vi "Color_Project.vi"() -> ()   [LabVIEW 2013]
uses:
  leitura de dados txt control.ctl
  <vilib>/Utility/file.llb/Write To Spreadsheet File (DBL).vi
panel:
  out "L*a*b* 3":dbl[](array[numeric])
  in  "C0":dbl min=0.0 max=1.0
  in  "RMix1":dbl[](array[numeric])
  in  "Selected RGB":string="0"
  in  "RMix2":dbl[](array[numeric])
  in  "Reflectance":dbl[](array[numeric])
  in  "Tab Control":T1(tab)
  in  "Create reflectance":bool
  in  "Nome da cor":string
  in  "SaveReflectance":bool
  out "Reflectance graph":cluster{"Value":dbl[], dbl[]}(graph) caption="Espectro de reflectância selecionado"
  in  "CalculateColor":bool
  in  "SelectReflectance":bool
  out "CMF graph":cluster{"X":dbl[], "Y":dbl[]}[](graph)
  in  "Select Illuminant":T2
  in  "Color Matching Function":string(combo)
  out "Iluminante Graph":cluster{"Value":dbl[], "Value":dbl[]}[](graph)
  in  "780nm":dbl(slide)=0.05 min=0.01 max=0.99 scale=0.0..1.0 scale format="%1.3f"
  in  "700nm":dbl(slide)=0.05 min=0.01 max=0.99 scale=0.0..1.0 scale format="%1.3f"
  in  "650nm":dbl(slide)=0.05 min=0.01 max=0.99 scale=0.0..1.0 scale format="%1.3f"
  in  "575nm":dbl(slide)=0.05 min=0.01 max=0.99 scale=0.0..1.0 scale format="%1.3f"
  in  "550nm":dbl(slide)=0.05 min=0.01 max=0.99 scale=0.0..1.0 scale format="%1.3f"
  in  "525nm":dbl(slide)=0.05 min=0.01 max=0.99 scale=0.0..1.0 scale format="%1.3f"
  in  "500nm":dbl(slide)=0.05 min=0.01 max=0.99 scale=0.0..1.0 scale format="%1.3f"
  in  "600nm":dbl(slide)=0.05 min=0.01 max=0.99 scale=0.0..1.0 scale format="%1.3f"
  in  "450nm":dbl(slide)=0.05 min=0.01 max=0.99 scale=0.0..1.0 scale format="%1.3f"
  in  "380nm":dbl(slide)=0.05 min=0.01 max=0.99 scale=0.0..1.0 scale format="%1.3f"
  out "Color":u32(colorbox)
  out "RGB":dbl[](array[numeric])
  out "XYZ":dbl[](array[numeric])
  out "RGB255":u32[](array[numeric]) caption="RGB"
  in  "Tab Control 3":enum32{"Misturar", "Estatísticas"}(tab)
  out "ColorRM":cluster{"Value":dbl[], "Mixtured colors":dbl[]}(graph) caption="Gráfico da reflectância das cores misturadas"
  in  "MixColors":bool
  in  "Selecione a concentração da cor 1":dbl(slide) scale=0.0..1.0 scale format="%#.4g"
  out "2000":dbl caption="Diferença: Cor 1 - Cor misturada"
  out "CD2-M":dbl caption="Diferença: Cor 2 - Cor misturada"
  out "L*a*b* MixedColor":dbl[](array[numeric]) caption="L*a*b* mixtura"
  out "L*a*b*":dbl[](array[numeric]) caption="L*a*b* cor 1"
  out "L*a*b* 2":dbl[](array[numeric]) caption="L*a*b* cor 2"
  out "Cor complementar":u32(colorbox)
  out "MixedColors":u32(colorbox) caption="Cor resultante"
  out "ColorR2":cluster{"Value":dbl[], "Mixtured colors":dbl[]}(graph) caption="Gráfico de reflectância da cor 2"
  out "ColorR1":cluster{"Value":dbl[], "Mixtured colors":dbl[]}(graph) caption="Gráfico de reflectância da cor 1"
  out "Color2":u32(colorbox) caption="Cor selecionada"
  out "Color1":u32(colorbox) caption="Cor selecionada"
  in  "SelectColor2":bool
  in  "SelectColor1":bool
  in  "Color Matching Function 2":string(combo) caption="Selecione o CMF"
  in  "SelectIlluminant2":T2 caption="Selecione o iluminante"
  out "Color1Complementar":u32(colorbox) caption="Cor complementar"
  out "Cor complementar  2":u32(colorbox) caption="Cor complementar"
  in  "SelectColor2":bool
  in  "SelectColor1":bool
  in  "Tab Control 2":enum32{"L*", "a*", "b*"}(tab)
  out "Componente L*":cluster{"X":dbl[], "L*a*b intermediary":dbl[]}(graph)
  out "Componente a*":cluster{"X":dbl[], "L*a*b intermediary":dbl[]}(graph)
  out "Componente b*":cluster{"X":dbl[], "L*a*b intermediary":dbl[]}(graph)
  in  "Color Matching Function 3":string(combo) caption="Selecione o CMF"
  in  "SelectIlluminant2 2":T2 caption="Selecione o iluminante"
  in  "Colors":u32[](array[colorbox])
  out "Espectros de reflectância referentes as cores intermediárias obtidas":cluster{"X":dbl[], "Y":dbl[]}[](graph)
  in  "MixByConcentration":bool
  in  "Mixed":dbl[](array[numeric])
  in  "MixByColorDifference":bool
  out "Color1 2":u32
  out "Color2 2":u32
  in  "C1":dbl=0.1 min=0.0 max=1.0
  in  "DeltaLabel":string[](array[string]) caption="Delta E"
  in  "ConcentrationLabel":string[](array[string]) caption="Concentração"
  out "teste":i32[](array[numeric])
  out "IL Table":string[][](array[string])
  out "ILCols":i32
  out "ILRows":i32
  out "Selected illuminant value":dbl[](array[numeric])
  out "Is CMF selected?":bool
  out "Is illuminant selected?":bool
  out "CMF Table":string[][](array[string])
  out "NeedInterpolation?":bool
  out "WhiteReference":i32[](array[numeric])
  out "Intepoled iluminants":dbl[][](array[numeric])
  out "Selected\nCMF":dbl[][](array[numeric])
  out "cmf Index":dbl
  out "CMFCols":i32
  out "CMFRows":i32
  out "LambdaInterval":dbl[](array[numeric])
  out "Selected illuminant index":dbl
  out "Selected illuminant NV":cluster{"Value":string, dbl[]}
  # "Primeira etapa - Seleção da iluminação desejada"
  # "Segunda etapa - Seleção do estímulo ocular do observador"
  # "Terceira etapa - Seleção ou criação de espectros de reflectância"
  # "Selecione o CMF"
  # "Selecione o iluminante"
  # "Etapa final - Calcular cor referente aos espectros"
  # "Sistema para criação de espectros de reflectância"
  # "Etapa básica - Seleção de iluminação e estímulos oculares"
  # "Etapa final - Calcular a mistura das cores e dosar a concentração da cor referência"
  # "Segunda etapa - Selecionar as cores desejadas para efetuar a mistura"
  # "Desvios de cor"
  # "Coordenadas de cor"
  # "Nesta seção serão avaliadas diferentes maneiras para misturas de cores:\n1 - Por variação de concentração\n2 - Por variação de desvio de cor"
  # "Análise de variação das componentes L*a*b* das cores geradas"
  # "Seleção de componentes"
  # "Seleção do tipo da mistura a ser efetuado"
  # "Representação das cores intermediárias gerada a partir\ndas misturas,e seus respectivos desvios e concentrações"
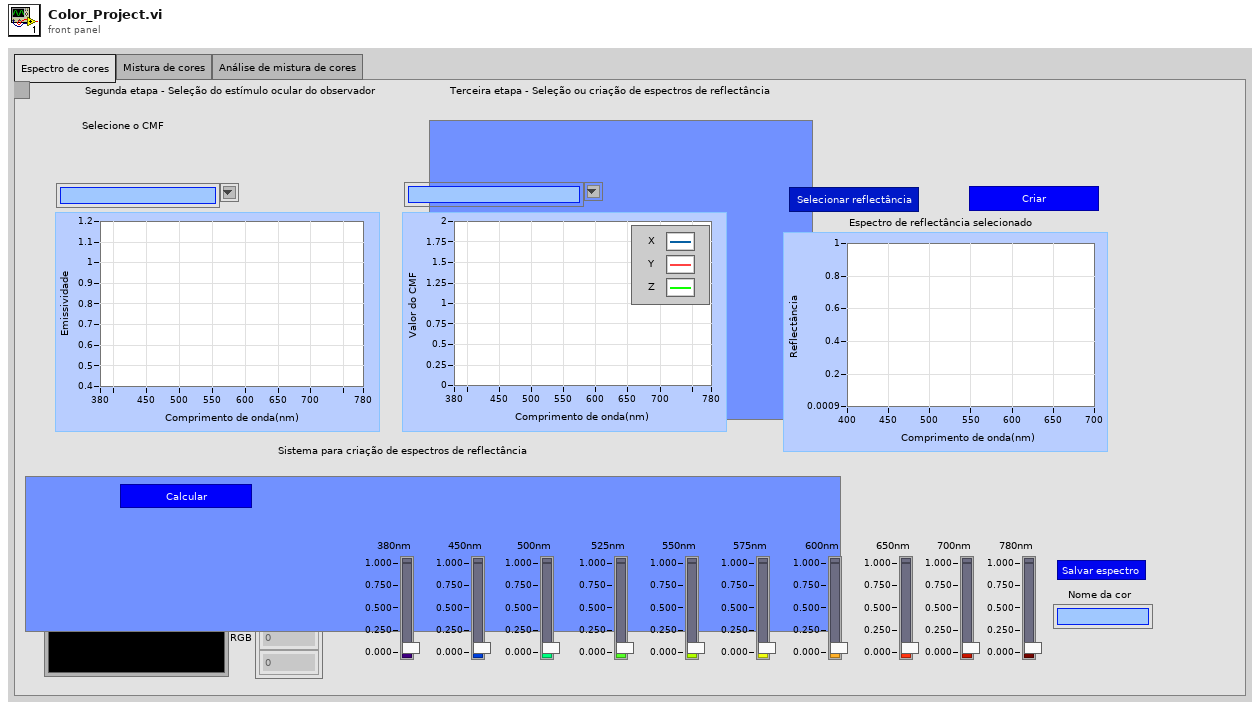
[diagram p1: front panel]
types:
  T1 = enum32{"Espectro de cores", "Mistura de cores", "Análise de mistura de cores"}
  T2 = typedef "leitura de dados txt control.ctl" = string
  T3 = cluster{"Value":cluster{"Value":string, dbl[]}, "Selected RGB":string, "Value":dbl[][]}
  T4 = cluster{"Color":u32, "RGB":dbl[], "L*a*b*":dbl[], "XYZ":dbl[]}
  T5 = cluster{cluster{i32[], dbl[]}, cluster{i32[], dbl[]}, cluster{i32[], dbl[]}}
  T6 = cluster{cluster{"X":dbl[], "L*a*b intermediary":dbl[]}, cluster{"X":dbl[], "L*a*b intermediary":dbl[]}, cluster{"X":dbl[], "L*a*b intermediary":dbl[]}}
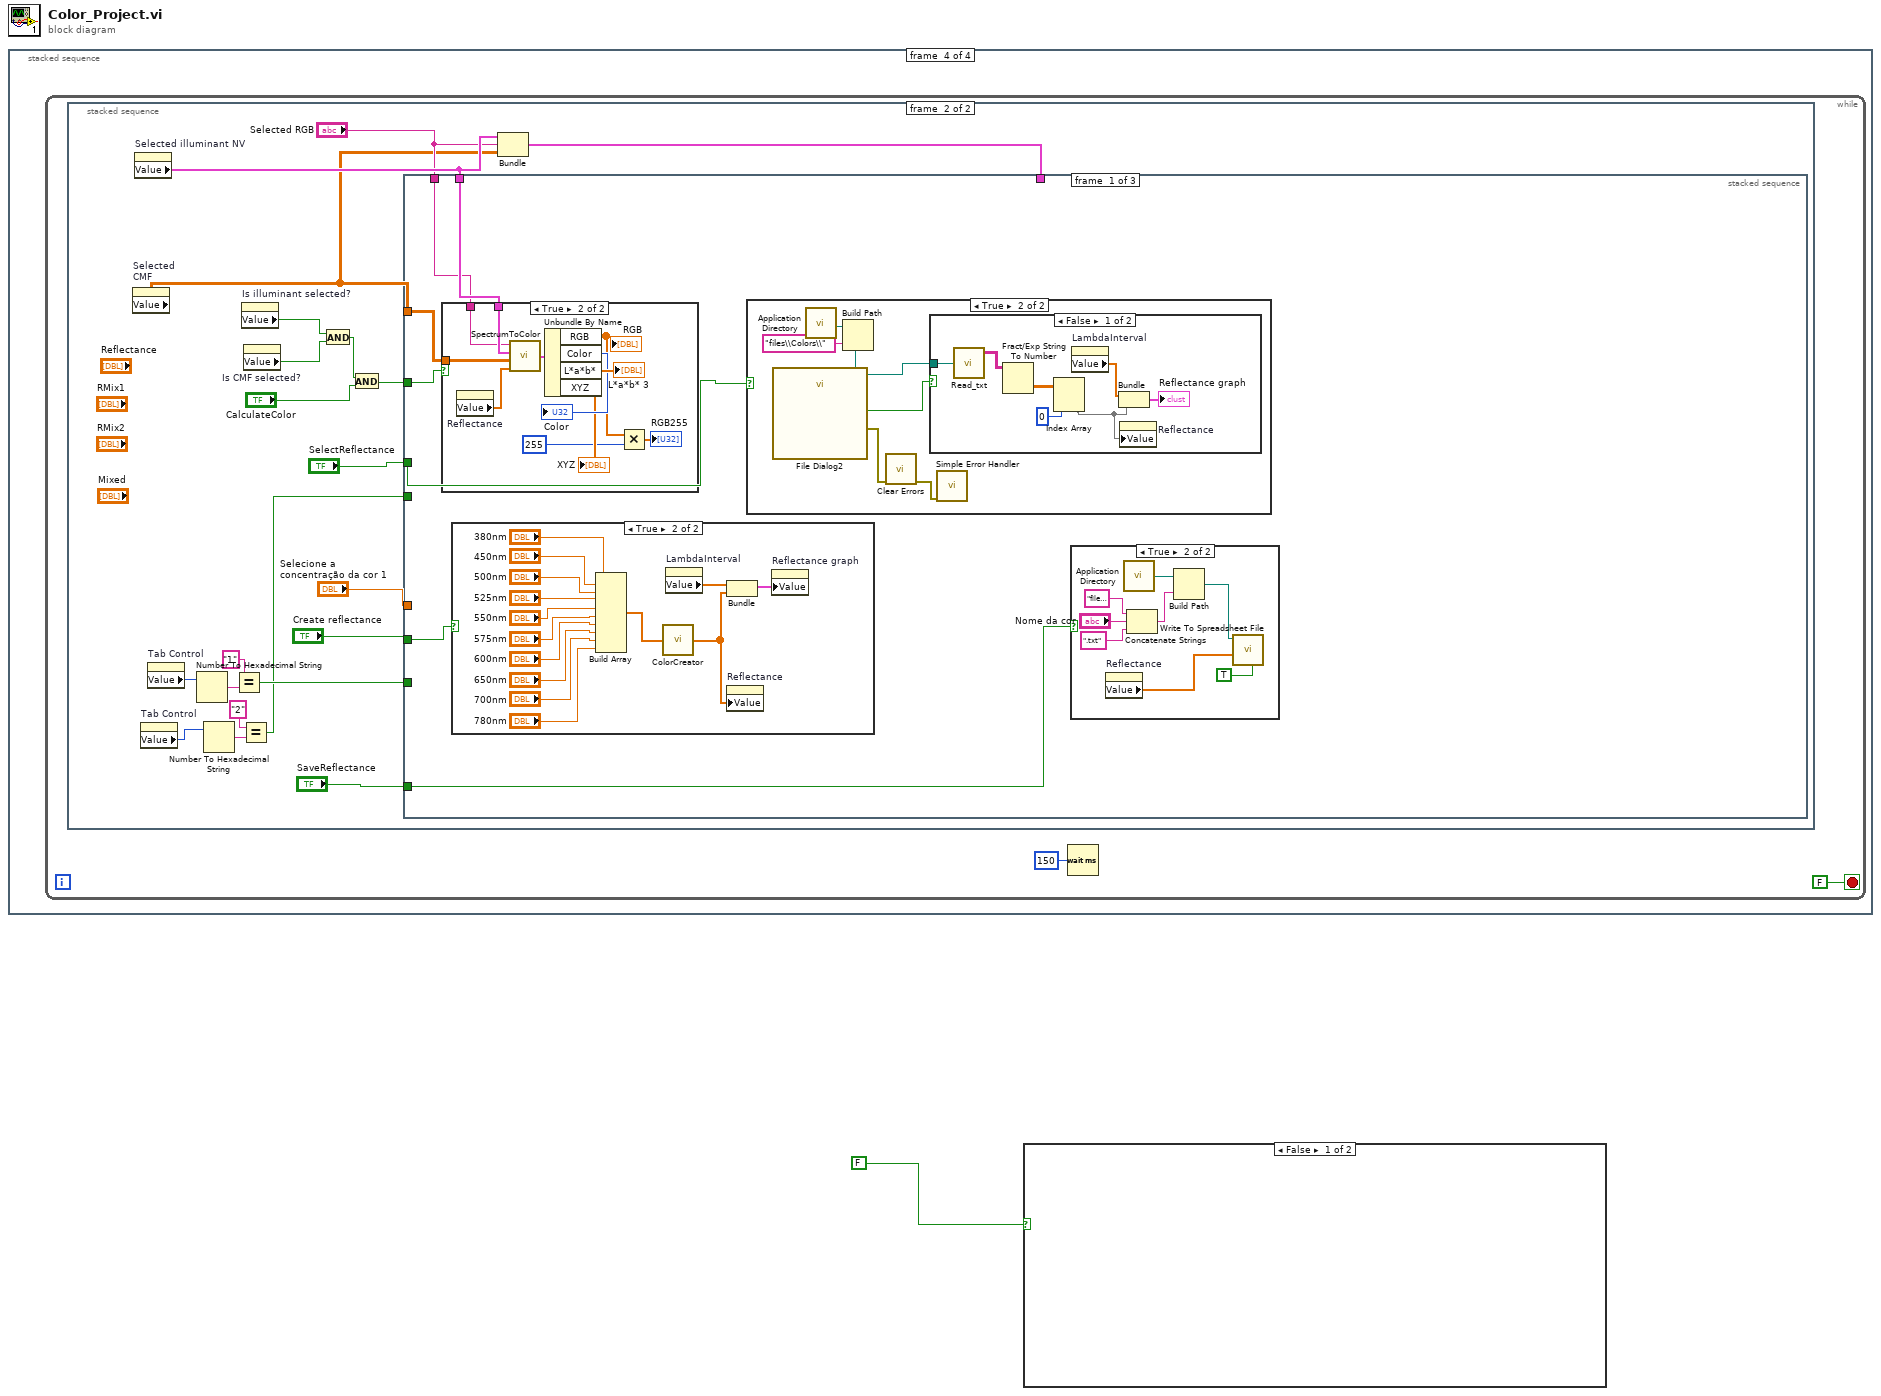
[diagram p0: block diagram]
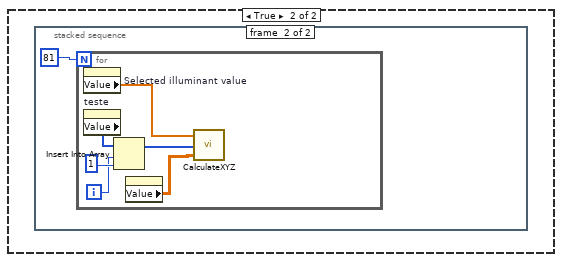
[diagram p2: hidden frame]
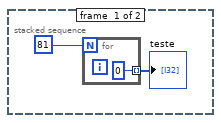
[diagram p3: hidden frame]
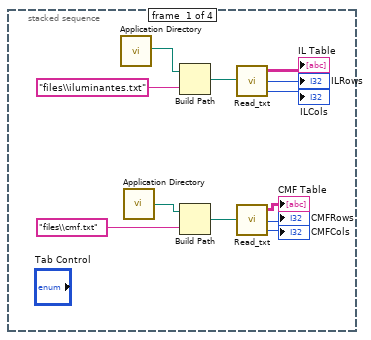
[diagram p4: hidden frame]
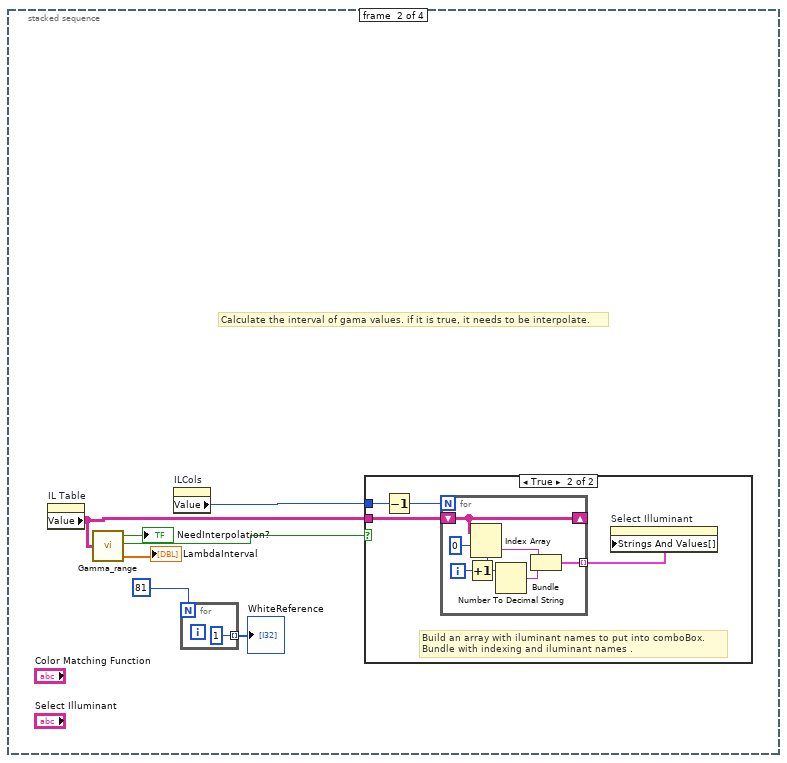
[diagram p5: hidden frame]
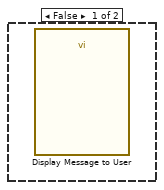
[diagram p6: hidden frame]
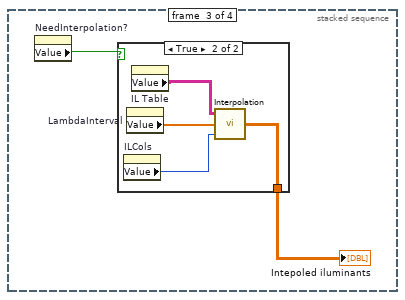
[diagram p7: hidden frame]
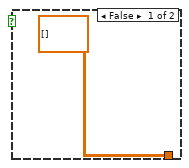
[diagram p8: hidden frame]
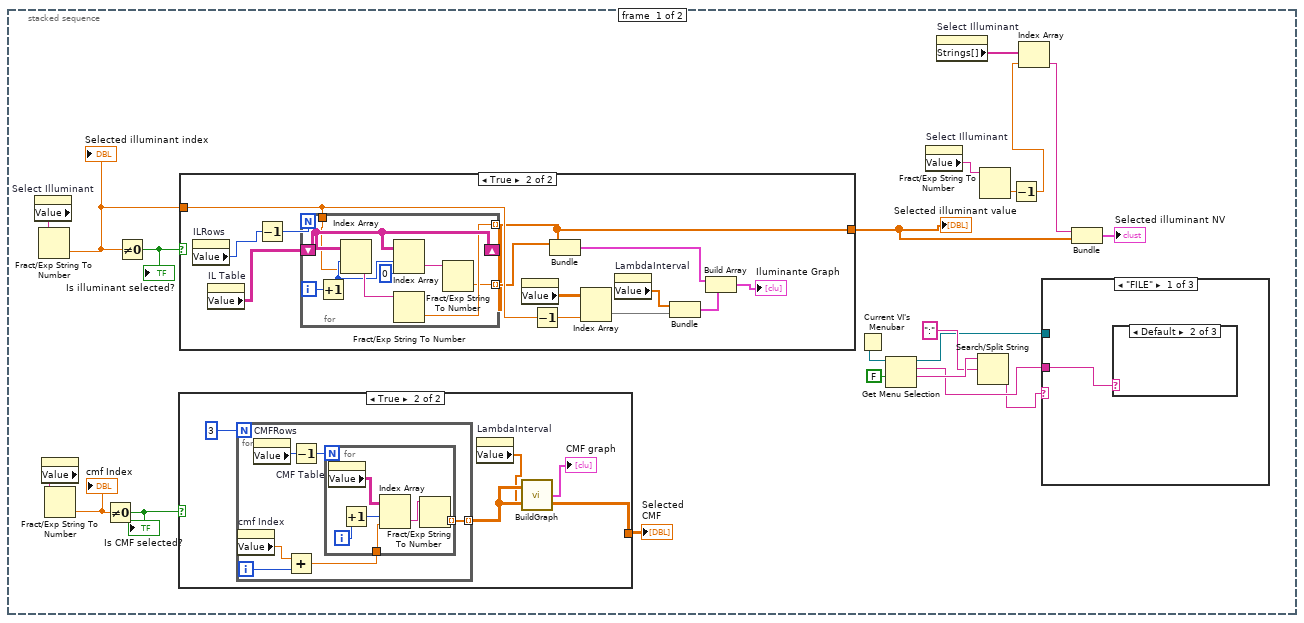
[diagram p9: hidden frame]
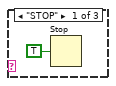
[diagram p10: hidden frame]
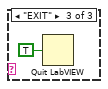
[diagram p11: hidden frame]
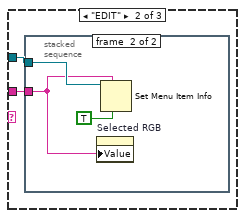
[diagram p12: hidden frame]
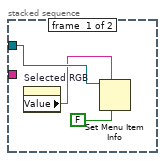
[diagram p13: hidden frame]
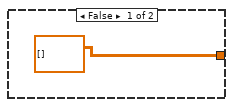
[diagram p15: hidden frame]
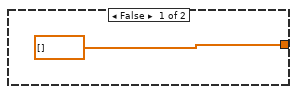
[diagram p16: hidden frame]
diagram:
  n1 = stacked-sequence {
    frame #0 {
      n2 = call <vilib>:"Application Directory.vi"() -> ("Application Directory"=w3:path)
      n3 = call <vilib>:"Application Directory.vi"() -> ("Application Directory"=w2:path)
      n4 = Build Path(base path=w3, name or relative path="files\\iluminantes.txt") -> (appended path=w5:path)
      n5 = Build Path(base path=w2, name or relative path="files\\cmf.txt") -> (appended path=w4:path)
      n6 = call "Read_txt.vi"("file path (dialog if empty)"=w5) -> ("Elements"=→"IL Table":string[][], "Rows"=→"ILRows":i32, "Cols"=→"ILCols":i32)
      n7 = call "Read_txt.vi"("file path (dialog if empty)"=w4) -> ("Elements"=→"CMF Table":string[][], "Rows"=→"CMFRows":i32, "Cols"=→"CMFCols":i32)
    }
    frame #1 {
      # "Calculate the interval of gama values. if it is true, it needs to be interpolate."
      n8 = property on="IL Table" class="Arr (strict)"() -> ("Value"=w15:string[][])  [unwired: 2 in, 2 out]
      n9 = call "Gamma_range.vi"("Illuminant Table"=w15) -> ("Interpolate"=→"NeedInterpolation?":bool, "In range?"=w17:bool, "GammaInterval"=→"LambdaInterval":dbl[])
      n10 = property on="ILCols" class="DigNum (strict)"() -> ("Value"=w18:i32)  [unwired: 2 in, 2 out]
      n11 = for {
        N: 81 -> [_]
        tunnel: [1] -> w19 mode=indexing
      }
      "WhiteReference" <- w19
      n12 = case shown="True" w17 {
        tunnel: w15 -> [_ w21]
        tunnel: w18 -> [_ w22]
        frame False {
          n13 = call "Display Message to User"() -> ()  [unwired: 10 in, 2 out]
        }
        frame True {
          # "Build an array with iluminant names to put into comboBox.\nBundle with indexing and iluminant names ."
          n14 = Decrement(x=w22) -> (x-1=w24:i32)
          n15 = for {
            N: w24 -> [_]
            shift-right: [w29] -> _
            shift-left: w21 -> [w29]
            tunnel: [w25] -> w23 mode=indexing
            i -> [w31]
            n16 = Increment(x=w31) -> (x+1=w28:i32)
            n17 = Index Array(array=w29, index (row)=0, index (col)=w28) -> (element=w26:string)
            n18 = Number To Decimal String(number=w28) -> (decimal integer string=w27:string)  [unwired: 1 in]
            n19 = Bundle("String"=w26, w27) -> (w25:cluster{"String":string, string})  [unwired: 1 in]
          }
          n20 = property on="Select Illuminant" class="CmbBox (strict)"("Strings And Values[]"=w23) -> ()  [unwired: 2 in, 2 out]
        }
      }
    }
    frame #2 {
      n21 = property on="NeedInterpolation?" class="Bool (strict)"() -> ("Value"=w34:bool)  [unwired: 2 in, 2 out]
      n22 = case shown="True" w34 {
        tunnel: [dbl[][] [] w38] -> w33
        frame False {
        }
        frame True {
          n23 = property on="ILCols" class="DigNum (strict)"() -> ("Value"=w36:i32)  [unwired: 2 in, 2 out]
          n24 = property on="LambdaInterval" class="Arr (strict)"() -> ("Value"=w39:dbl[])  [unwired: 2 in, 2 out]
          n25 = property on="IL Table" class="Arr (strict)"() -> ("Value"=w37:string[][])  [unwired: 2 in, 2 out]
          n26 = call "Interpolation.vi"("Number of Columns"=w36, "Lambda Interval"=w39, "Illuminants"=w37) -> ("Interpolated"=w38:dbl[][])
        }
      }
      "Intepoled iluminants" <- w33
    }
    frame #3 {
      n27 = while {
        stop <- FALSE stop-if-true
        n28 = stacked-sequence {
          frame #0 {
            n29 = property on="Select Illuminant" class="CmbBox (strict)"() -> ("Value"=w58:T2)  [unwired: 2 in, 2 out]
            n30 = Fract/Exp String To Number(string=w58) -> (number=w57:dbl)  [unwired: 3 in, 1 out]
            "Selected illuminant index" <- w57
            n31 = property on="Color Matching Function" class="CmbBox"() -> ("Value"=w60:string)  [unwired: 2 in, 2 out]
            n32 = Fract/Exp String To Number(string=w60) -> (number=w61:dbl)  [unwired: 3 in, 1 out]
            "cmf Index" <- w61
            n33 = Not Equal To 0?(x=w61) -> (x != 0?=w59:bool)
            "Is CMF selected?" <- w59
            n34 = Not Equal To 0?(x=w57) -> (x != 0?=w62:bool)
            "Is illuminant selected?" <- w62
            n35 = case shown="True" w59 {
              tunnel: [dbl[][] [] w77] -> w56
              frame False {
              }
              frame True {
                n36 = for {
                  N: 3 -> [_]
                  tunnel: [w81] -> w77 mode=indexing
                  i -> [w83]
                  n37 = property on="cmf Index" class="DigNum (strict)"() -> ("Value"=w84:dbl)  [unwired: 2 in, 2 out]
                  n38 = property on="CMFRows" class="DigNum (strict)"() -> ("Value"=w80:i32)  [unwired: 2 in, 2 out]
                  n39 = Add(x=w84, y=w83) -> (x+y=w82:dbl)
                  n40 = Decrement(x=w80) -> (x-1=w79:i32)
                  n41 = for {
                    N: w79 -> [_]
                    tunnel: w82 -> [w89]
                    tunnel: [w85] -> w81 mode=indexing
                    i -> [w88]
                    n42 = property on="CMF Table" class="Arr (strict)"() -> ("Value"=w90:string[][])  [unwired: 2 in, 2 out]
                    n43 = Increment(x=w88) -> (x+1=w87:i32)
                    n44 = Index Array(array=w90, index (row)=w87, index (col)=w89) -> (element=w86:string)
                    n45 = Fract/Exp String To Number(string=w86) -> (number=w85:dbl)  [unwired: 3 in, 1 out]
                  }
                }
                n46 = property on="LambdaInterval" class="Arr (strict)"() -> ("Value"=w76:dbl[])  [unwired: 2 in, 2 out]
                n47 = call "BuildGraph.vi"("X"=w76, "Y"=w77) -> ("Graph"=→"CMF graph":cluster{"X":dbl[], "Y":dbl[]}[])
              }
            }
            "Selected\nCMF" <- w56
            n48 = case shown="True" w62 {
              tunnel: w57 -> [_ w101]
              tunnel: [dbl[] [] w95] -> w55
              frame False {
              }
              frame True {
                n49 = property on="ILRows" class="DigNum (strict)"() -> ("Value"=w94:i32)  [unwired: 2 in, 2 out]
                n50 = property on="IL Table" class="Arr (strict)"() -> ("Value"=w93:string[][])  [unwired: 2 in, 2 out]
                n51 = Decrement(x=w94) -> (x-1=w104:i32)
                n52 = for {
                  N: w104 -> [_]
                  shift-right: [w112] -> _
                  shift-left: w93 -> [w112]
                  tunnel: w101 -> [w105]
                  tunnel: [w107] -> w95 mode=indexing
                  tunnel: [w106] -> w97 mode=indexing
                  i -> [w113]
                  n53 = Increment(x=w113) -> (x+1=w108:i32)
                  n54 = Index Array(array=w112, index (row)=w108, index (col)=w105) -> (element=w109:string)
                  n55 = Index Array(array=w112, index (row)=w108, index (col)=0 ("disabled index (col)")) -> (element=w110:string)
                  n56 = Fract/Exp String To Number(string=w109) -> (number=w107:dbl)  [unwired: 3 in, 1 out]
                  n57 = Fract/Exp String To Number(string=w110) -> (number=w106:dbl)  [unwired: 3 in, 1 out]
                }
                n58 = property on="Intepoled iluminants" class="Arr (strict)"() -> ("Value"=w99:dbl[][])  [unwired: 2 in, 2 out]
                n59 = Decrement(x=w101) -> (x-1=w100:dbl)
                n60 = Bundle(w97, w95) -> (w102:cluster{dbl[], dbl[]})  [unwired: 1 in]
                n61 = Index Array(array=w99, index (col)=w100) -> (element=w96:dbl[])  [unwired: 1 in]
                n62 = property on="LambdaInterval" class="Arr (strict)"() -> ("Value"=w98:dbl[])  [unwired: 2 in, 2 out]
                n63 = Bundle("Value"=w98, "Value"=w96) -> (w103:cluster{"Value":dbl[], "Value":dbl[]})  [unwired: 1 in]
                n64 = Build Array(w102, w103) -> (→"Iluminante Graph":cluster{"Value":dbl[], "Value":dbl[]}[])
              }
            }
            "Selected illuminant value" <- w55
            n65 = Current VI's Menubar() -> (w42:refnum<k9>)
            n66 = Get Menu Selection(0:w42, 2:FALSE ("block menu (F)")) -> (5:w45:refnum<k9>, 6:w44:string, 7:w47:string)  [unwired: 2 in, 2 out]
            n67 = property on="Select Illuminant" class="CmbBox (strict)"() -> ("Value"=w51:T2)  [unwired: 2 in, 2 out]
            n68 = property on="Select Illuminant" class="CmbBox (strict)"() -> ("Strings[]"=w53:string[])  [unwired: 2 in, 2 out]
            n69 = Search/Split String(string=w47, search string/char (-)=":") -> (substring before match=w43:string)  [unwired: 1 in, 2 out]
            n70 = Fract/Exp String To Number(string=w51) -> (number=w50:dbl)  [unwired: 3 in, 1 out]
            n71 = Decrement(x=w50) -> (x-1=w49:dbl)
            n72 = Index Array(array=w53, index=w49) -> (element=w52:string)
            n73 = case shown="\"FILE\"" w43 {
              tunnel: w45 -> [_ w67 _]
              tunnel: w44 -> [w63 w66 _]
              frame "FILE" {
                n74 = case shown="Default" w63 {
                  frame "STOP" {
                    n75 = Stop(stop? (T)=TRUE) -> ()
                  }
                  frame Default {
                  }
                  frame "EXIT" {
                    n76 = Quit LabVIEW(quit? (T)=TRUE) -> ()
                  }
                }
              }
              frame "EDIT" {
                n77 = stacked-sequence {
                  tunnel: w67 -> [w70 w73]
                  tunnel: w66 -> [_ w72]
                  frame #0 {
                    n78 = property on="Selected RGB" class="Str"() -> ("Value"=w68:string)  [unwired: 2 in, 2 out]
                    n79 = Set Menu Item Info(6:FALSE ("enabled"), 7:w68, 11:w70) -> ()  [unwired: 4 in, 2 out]
                  }
                  frame #1 {
                    n80 = property on="Selected RGB" class="Str"("Value"=w72) -> ()  [unwired: 2 in, 2 out]
                    n81 = Set Menu Item Info(6:TRUE ("enabled"), 7:w72, 11:w73) -> ()  [unwired: 4 in, 2 out]
                  }
                }
              }
              frame Default {
              }
            }
            n82 = Bundle(w52, w55) -> (→"Selected illuminant NV":cluster{string, dbl[]})  [unwired: 1 in]
          }
          frame #1 {
            n83 = property on="Selected\nCMF" class="Arr (strict)"() -> ("Value"=w125:dbl[][])  [unwired: 2 in, 2 out]
            n84 = property on="Selected illuminant NV" class="Clust (strict)"() -> ("Value"=w127:cluster{"Value":string, dbl[]})  [unwired: 2 in, 2 out]
            n85 = property on="Tab Control" class="TabCtl (strict)"() -> ("Value"=w118:T1)  [unwired: 2 in, 2 out]
            n86 = property on="Tab Control" class="TabCtl (strict)"() -> ("Value"=w121:T1)  [unwired: 2 in, 2 out]
            n87 = Number To Hexadecimal String(2:w121) -> (0:w122:string)  [unwired: 1 in]
            n88 = Number To Hexadecimal String(2:w118) -> (0:w119:string)  [unwired: 1 in]
            n89 = Equal?(x="1", y=w122) -> (x = y?=w120:bool)
            n90 = Equal?(x="2", y=w119) -> (x = y?=w116:bool)
            n91 = property on="Is illuminant selected?" class="Bool (strict)"() -> ("Value"=w132:bool)  [unwired: 2 in, 2 out]
            n92 = property on="Is CMF selected?" class="Bool (strict)"() -> ("Value"=w133:bool)  [unwired: 2 in, 2 out]
            n93 = And(x=w132, y=w133) -> (x .and. y?=w114:bool)
            n94 = And(x=w114, y="CalculateColor") -> (x .and. y?=w131:bool)
            n95 = Bundle("Value"=w127, "Selected RGB"="Selected RGB", "Value"=w125) -> (w124:T3)  [unwired: 1 in]
            n96 = stacked-sequence {
              tunnel: w127 -> [w139 w191 w250]
              tunnel: w125 -> [w138 w190 w249]
              tunnel: w131 -> [w137 _ _]
              tunnel: "SelectReflectance" -> [w141 _ _]
              tunnel: "Create reflectance" -> [w140 _ _]
              tunnel: "Selected RGB" -> [w136 w192 w251]
              tunnel: "Selecione a concentração da cor 1" -> [_ w193 _]
              tunnel: "SaveReflectance" -> [w135 _ _]
              tunnel: w124 -> [_ _ w248]
              tunnel: w120 -> [_ w189 _]
              tunnel: w116 -> [_ _ w247]
              frame #0 {
                n97 = case shown="True" w137 {
                  tunnel: w139 -> [_ w159]
                  tunnel: w138 -> [_ w158]
                  tunnel: w136 -> [_ w156]
                  frame False {
                  }
                  frame True {
                    n98 = property on="Reflectance" class="Arr (strict)"() -> ("Value"=w157:dbl[])  [unwired: 2 in, 2 out]
                    n99 = call "SpectrumToColor.vi"("Reflectance"=w157, "CMF"=w158, "Illuminant"=w159, "Selected RGB"=w156) -> ("Color,XYZ,RGB,Lab"=w160:T4)
                    n100 = Unbundle By Name(w160) -> ("RGB"=w150:dbl[], "Color"=→"Color":u32, "L*a*b*"=→"L*a*b* 3":dbl[], "XYZ"=→"XYZ":dbl[])
                    "RGB" <- w150
                    n101 = Multiply(x=w150, y=255) -> (x*y=→"RGB255":dbl[])
                  }
                }
                n102 = case shown="True" w140 {
                  frame False {
                  }
                  frame True {
                    n103 = Build Array("380nm", "450nm", "500nm", "525nm", "550nm", "575nm", "600nm", "650nm", "700nm", "780nm") -> (w164:dbl[])
                    n104 = call "ColorCreator.vi"("Reflectance values"=w164) -> ("Spectrum"=w161:dbl[])
                    n105 = property on="LambdaInterval" class="Arr (strict)"() -> ("Value"=w162:dbl[])  [unwired: 2 in, 2 out]
                    n106 = Bundle("Value"=w162, "Spectrum"=w161) -> (w163:cluster{"Value":dbl[], "Spectrum":dbl[]})  [unwired: 1 in]
                    n107 = property on="Reflectance" class="Arr (strict)"("Value"=w161) -> ()  [unwired: 2 in, 2 out]
                    n108 = property on="Reflectance graph" class="XYGraph (strict)"("Value"=w163) -> ()  [unwired: 2 in, 2 out]
                  }
                }
                n109 = case shown="True" w141 {
                  frame False {
                  }
                  frame True {
                    n110 = call <vilib>:"Application Directory.vi"() -> ("Application Directory"=w180:path)
                    n111 = Build Path(base path=w180, name or relative path="files\\Colors\\") -> (appended path=w179:path)
                    n112 = call "File Dialog2"("start path"=w179) -> ("selected path"=w177:path, "cancelled"=w178:bool, "error out"=w176:errorcluster)  [unwired: 11 in, 1 out]
                    n113 = call <vilib>:"Clear Errors.vi"("error in (no error)"=w176) -> ("error out"=w175:errorcluster)  [unwired: 6 in]
                    n114 = case shown="False" w178 {
                      tunnel: w177 -> [w183 _]
                      frame False {
                        n115 = call "Read_txt.vi"("file path (dialog if empty)"=w183) -> ("Elements"=w188:string[][])  [unwired: 2 out]
                        n116 = Fract/Exp String To Number(string=w188) -> (number=w187:dbl[][])  [unwired: 3 in, 1 out]
                        n117 = Index Array(array=w187, index (col)=0 ("index (row)")) -> (element=w182:dbl[])  [unwired: 1 in]
                        n118 = property on="LambdaInterval" class="Arr (strict)"() -> ("Value"=w185:dbl[])  [unwired: 2 in, 2 out]
                        n119 = Bundle("Value"=w185, w182) -> (→"Reflectance graph":cluster{"Value":dbl[], dbl[]})  [unwired: 1 in]
                        n120 = property on="Reflectance" class="Arr (strict)"("Value"=w182) -> ()  [unwired: 2 in, 2 out]
                      }
                      frame True {
                        n121 = call "Display Message to User2"() -> ()  [unwired: 10 in, 2 out]
                      }
                    }
                    n122 = call <vilib>:"Simple Error Handler.vi"("error in (no error)"=w175) -> ()  [unwired: 4 in, 5 out]
                  }
                }
                n123 = case shown="True" w135 {
                  frame False {
                  }
                  frame True {
                    n124 = property on="Reflectance" class="Arr (strict)"() -> ("Value"=w147:dbl[])  [unwired: 2 in, 2 out]
                    n125 = call <vilib>:"Application Directory.vi"() -> ("Application Directory"=w149:path)
                    n126 = Concatenate Strings("files\\Colors\\" ("name or relative path"), "Nome da cor", ".txt") -> (w143:string)
                    n127 = Build Path(base path=w149, name or relative path=w143) -> (appended path=w148:path)
                    n128 = call-poly <vilib>:"Write To Spreadsheet File.vi"("transpose? (no:F)"=TRUE, "1D data"=w147, "file path (dialog if empty)"=w148) -> ()  [unwired: 5 in, 1 out]
                  }
                }
              }
              frame #1 {
                n129 = case shown="True" w189 {
                  tunnel: w193 -> [_ w208]
                  tunnel: w192 -> [_ w207]
                  tunnel: w191 -> [_ w206]
                  tunnel: w190 -> [_ w205]
                  frame False {
                  }
                  frame True {
                    n130 = property on="Color Matching Function" class="CmbBox"("Value"="Color Matching Function 2") -> ()  [unwired: 2 in, 2 out]
                    n131 = case shown="True" "MixColors" {
                      tunnel: w208 -> [_ w223]
                      frame False {
                      }
                      frame True {
                        n132 = property on="RMix2" class="Arr (strict)"() -> ("Value"=w224:dbl[])  [unwired: 2 in, 2 out]
                        n133 = property on="RMix1" class="Arr (strict)"() -> ("Value"=w213:dbl[])  [unwired: 2 in, 2 out]
                        n134 = call "ColorMixture.vi"("Concentration1"=w223, "Reflectance spectrum 2"=w224, "Reflectance spectrum"=w213) -> ("Mixtured colors"=w218:dbl[])  [unwired: 1 in]
                        n135 = property on="Selected illuminant NV" class="Clust (strict)"() -> (error out=w216:errorcluster, "Value"=w222:cluster{"Value":string, dbl[]})  [unwired: 2 in, 1 out]
                        n136 = property on="Selected\nCMF" class="Arr (strict)"() -> ("Value"=w221:dbl[][])  [unwired: 2 in, 2 out]
                        n137 = property on="LambdaInterval" class="Arr (strict)"() -> ("Value"=w219:dbl[])  [unwired: 2 in, 2 out]
                        n138 = property on="Selected RGB" class="Str"(error in=w216) -> ("Value"=w215:string)  [unwired: 1 in, 2 out]
                        n139 = call "SpectrumToColor.vi"("Reflectance"=w218, "CMF"=w221, "Illuminant"=w222, "Selected RGB"=w215) -> ("Color,XYZ,RGB,Lab"=w220:T4)
                        n140 = Bundle("Value"=w219, "Mixtured colors"=w218) -> (→"ColorRM":cluster{"Value":dbl[], "Mixtured colors":dbl[]})  [unwired: 1 in]
                        n141 = Unbundle By Name(w220) -> ("Color"=w210:u32, "L*a*b*"=→"L*a*b* MixedColor":dbl[], "RGB"=w212:dbl[])
                        "MixedColors" <- w210
                        n142 = call "RGBtoComplementar.vi"("RGB"=w212) -> ("Complementar"=→"Cor complementar":u32)
                        n143 = property on="Selecione a concentração da cor 1" class="Slide (strict)"("Fill Color"=w210) -> ()  [unwired: 2 in, 2 out]
                      }
                    }
                    n144 = case shown="True" "SelectColor1" {
                      tunnel: w207 -> [_ w245]
                      tunnel: w206 -> [_ w244]
                      tunnel: w205 -> [_ w243]
                      frame False {
                      }
                      frame True {
                        n145 = call "SelectColor.vi"("CMF"=w243, "Illuminant"=w244, "Selected RGB"=w245) -> ("Reflectance"=w238:dbl[], "Color,XYZ,RGB,Lab"=w242:T4)
                        n146 = property on="RMix1" class="Arr (strict)"("Value"=w238) -> ()  [unwired: 2 in, 2 out]
                        n147 = property on="LambdaInterval" class="Arr (strict)"() -> ("Value"=w240:dbl[])  [unwired: 2 in, 2 out]
                        n148 = Unbundle By Name(w242) -> ("L*a*b*"=→"L*a*b*":dbl[], "Color"=→"Color1":u32, "RGB"=w237:dbl[])
                        n149 = Bundle("Value"=w240, "Reflectance"=w238) -> (→"ColorR1":cluster{"Value":dbl[], "Reflectance":dbl[]})  [unwired: 1 in]
                        n150 = call "RGBtoComplementar.vi"("RGB"=w237) -> ("Complementar"=→"Color1Complementar":u32)
                      }
                    }
                    n151 = case shown="True" "SelectColor2" {
                      tunnel: w207 -> [_ w235]
                      tunnel: w206 -> [_ w234]
                      tunnel: w205 -> [_ w233]
                      frame False {
                      }
                      frame True {
                        n152 = call "SelectColor.vi"("CMF"=w233, "Illuminant"=w234, "Selected RGB"=w235) -> ("Reflectance"=w228:dbl[], "Color,XYZ,RGB,Lab"=w231:T4)
                        n153 = Unbundle By Name(w231) -> ("L*a*b*"=→"L*a*b* 2":dbl[], "Color"=→"Color2":u32, "RGB"=w226:dbl[])
                        n154 = property on="RMix2" class="Arr (strict)"("Value"=w228) -> ()  [unwired: 2 in, 2 out]
                        n155 = property on="LambdaInterval" class="Arr (strict)"() -> ("Value"=w229:dbl[])  [unwired: 2 in, 2 out]
                        n156 = Bundle("Value"=w229, "Reflectance"=w228) -> (→"ColorR2":cluster{"Value":dbl[], "Reflectance":dbl[]})  [unwired: 1 in]
                        n157 = call "RGBtoComplementar.vi"("RGB"=w226) -> ("Complementar"=→"Cor complementar  2":u32)
                      }
                    }
                    n158 = property on="Select Illuminant" class="CmbBox (strict)"("Value"="SelectIlluminant2") -> ()  [unwired: 2 in, 2 out]
                    n159 = property on="L*a*b* MixedColor" class="Arr (strict)"() -> ("Value"=w199:dbl[])  [unwired: 2 in, 2 out]
                    n160 = property on="L*a*b*" class="Arr (strict)"() -> ("Value"=w201:dbl[])  [unwired: 2 in, 2 out]
                    n161 = property on="L*a*b* 2" class="Arr (strict)"() -> ("Value"=w200:dbl[])  [unwired: 2 in, 2 out]
                    n162 = Bundle("Value"=w200, "Value"=w199) -> (w196:cluster{"Value":dbl[], "Value":dbl[]})  [unwired: 1 in]
                    n163 = Bundle("Value"=w201, "Value"=w199) -> (w195:cluster{"Value":dbl[], "Value":dbl[]})  [unwired: 1 in]
                    n164 = call "DeltaE(2000).vi"("L*a*b Colors"=w196) -> ("Delta E"=→"CD2-M":dbl)
                    n165 = call "DeltaE(2000).vi"("L*a*b Colors"=w195) -> ("Delta E"=→"2000":dbl)
                  }
                }
              }
              frame #2 {
                n166 = case shown="True" w247 {
                  tunnel: w251 -> [_ w263]
                  tunnel: w250 -> [_ w262]
                  tunnel: w249 -> [_ w261]
                  tunnel: w248 -> [_ w260]
                  frame False {
                  }
                  frame True {
                    n167 = case shown="True" "MixByConcentration" {
                      tunnel: w263 -> [_ w389]
                      tunnel: w262 -> [_ w388]
                      tunnel: w261 -> [_ w387]
                      frame False {
                      }
                      frame True {
                        n168 = property on="LambdaInterval" class="Arr (strict)"() -> ("Value"=w385:dbl[])  [unwired: 2 in, 2 out]
                        n169 = for {
                          N: 11 -> [_]
                          tunnel: w389 -> [w399]
                          tunnel: w388 -> [w398]
                          tunnel: w387 -> [w397]
                          tunnel: [w395] -> w381 mode=indexing
                          tunnel: [w394] -> w386 mode=indexing
                          tunnel: [w393] -> w382 mode=indexing
                          tunnel: [w391] -> w375 mode=indexing
                          i -> [w392]
                          n170 = property on="RMix1" class="Arr (strict)"() -> ("Value"=w401:dbl[])  [unwired: 2 in, 2 out]
                          n171 = property on="RMix2" class="Arr (strict)"() -> ("Value"=w400:dbl[])  [unwired: 2 in, 2 out]
                          n172 = Divide(x=w392, y=10) -> (x/y=w393:dbl)
                          n173 = call "ColorMixture.vi"("Concentration1"=w393, "Reflectance spectrum 2"=w400, "Reflectance spectrum"=w401) -> ("Mixtured colors"=w394:dbl[])  [unwired: 1 in]
                          n174 = call "SpectrumToColor.vi"("Reflectance"=w394, "CMF"=w397, "Illuminant"=w398, "Selected RGB"=w399) -> ("Color,XYZ,RGB,Lab"=w396:T4)
                          n175 = Unbundle By Name(w396) -> ("Color"=w395:u32, "L*a*b*"=w391:dbl[])
                        }
                        n176 = call "BuildGraph.vi"("X"=w385, "Y"=w386) -> ("Graph"=w384:cluster{"X":dbl[], "Y":dbl[]}[])
                        n177 = property on="Espectros de reflectância referentes as cores intermediárias obtidas" class="XYGraph (strict)"("Value"=w384) -> ()  [unwired: 2 in, 2 out]
                        n178 = Number To Fractional String(number=w382, precision (6)=i16 2) -> (F-format string=w376:string[])  [unwired: 2 in]
                        n179 = property on="Colors" class="Arr (strict)"("Value"=w381) -> ()  [unwired: 2 in, 2 out]
                        n180 = call "LabConcentrationGraph.vi"("L*a*b*"=w375) -> ("L*a*b Variation"=w380:T5)
                        n181 = call "BuildDeltaString.vi"("L*a*b"=w375) -> ("DeltaEString"=w374:string[])
                        n182 = property on="ConcentrationLabel" class="Arr (strict)"("Value"=w376) -> ()  [unwired: 2 in, 2 out]
                        n183 = Unbundle(w380) -> (w379:cluster{i32[], dbl[]}, w378:cluster{i32[], dbl[]}, w377:cluster{i32[], dbl[]})
                        n184 = property on="DeltaLabel" class="Arr (strict)"("Value"=w374) -> ()  [unwired: 2 in, 2 out]
                        n185 = property on="Componente L*" class="XYGraph (strict)"("Value"=w379) -> ()  [unwired: 2 in, 2 out]
                        n186 = property on="Componente b*" class="XYGraph (strict)"("Value"=w378) -> ()  [unwired: 2 in, 2 out]
                        n187 = property on="Componente a*" class="XYGraph (strict)"("Value"=w377) -> ()  [unwired: 2 in, 2 out]
                      }
                    }
                    n188 = property on="RMix2" class="Arr (strict)"() -> (error out=w258:errorcluster, "Value"=w259:dbl[])  [unwired: 2 in, 1 out]
                    n189 = property on="Select Illuminant" class="CmbBox (strict)"("Value"="SelectIlluminant2 2") -> ()  [unwired: 2 in, 2 out]
                    n190 = property on="Color Matching Function" class="CmbBox"("Value"="Color Matching Function 3") -> ()  [unwired: 2 in, 2 out]
                    n191 = property on="Mixed" class="Arr (strict)"(error in=w258, "Value"=w259) -> ()  [unwired: 1 in, 2 out]
                    n192 = case shown="True" "SelectColor2" {
                      frame False {
                      }
                      frame True {
                        n193 = call "FileToDoubleArray.vi"() -> ("Reflectance"=w264:dbl[])
                        n194 = property on="RMix2" class="Arr (strict)"("Value"=w264) -> ()  [unwired: 2 in, 2 out]
                      }
                    }
                    n195 = case shown="True" "SelectColor1" {
                      frame False {
                      }
                      frame True {
                        n196 = call "FileToDoubleArray.vi"() -> ("Reflectance"=w265:dbl[])
                        n197 = property on="RMix1" class="Arr (strict)"("Value"=w265) -> ()  [unwired: 2 in, 2 out]
                      }
                    }
                    n198 = case shown="True" "MixByColorDifference" {
                      tunnel: w260 -> [_ w278]
                      frame False {
                      }
                      frame True {
                        n199 = property on="C0" class="DigNum (strict)"("Value"=0.0 ("C0")) -> ()  [unwired: 2 in, 2 out]
                        n200 = property on="C1" class="DigNum (strict)"("Value"=0.1 ("C1")) -> ()  [unwired: 2 in, 2 out]
                        n201 = flat-sequence {
                          tunnel: w278 -> [w291]
                          tunnel: [w289] -> w275
                          tunnel: [w288] -> w274
                          tunnel: [w287] -> w273
                          tunnel: [w286] -> w272
                          tunnel: [w285] -> w271
                          tunnel: [w284] -> w270
                          tunnel: [w283] -> w269
                          tunnel: [w282] -> w268
                          tunnel: [w281] -> w267
                          tunnel: [w279] -> w266
                          tunnel: w275 -> [w365]
                          tunnel: w274 -> [w366]
                          tunnel: w273 -> [w362]
                          tunnel: w272 -> [w361]
                          tunnel: w271 -> [w356]
                          tunnel: w270 -> [w355]
                          tunnel: w269 -> [w353]
                          tunnel: w268 -> [w349]
                          tunnel: w267 -> [w338]
                          tunnel: w266 -> [w333]
                          frame #0 {
                            # "dE"
                            n202 = property on="RMix1" class="Arr (strict)"() -> ("Value"=w285:dbl[])  [unwired: 2 in, 2 out]
                            n203 = property on="RMix2" class="Arr (strict)"() -> ("Value"=w284:dbl[])  [unwired: 2 in, 2 out]
                            n204 = call "SpectrumDeltaE.vi"("Iluminant - RGB - CMF"=w291, "Reflectance 2"=w284, "Reflectance 1"=w285) -> ("Color1"=w289:T4, "Delta E"=w292:dbl, "Color2"=w288:T4)  [unwired: 1 in]
                            n205 = Divide(x=w292, y=10.0) -> (x/y=w290:dbl)
                            n206 = for {
                              N: 9 -> [_]
                              tunnel: w285 -> [w303]
                              tunnel: w284 -> [w302]
                              tunnel: w291 -> [w301]
                              tunnel: w290 -> [w300]
                              tunnel: [w298] -> w286 mode=indexing
                              tunnel: [w297] -> w287 mode=indexing
                              tunnel: [w296] -> w283 mode=indexing
                              tunnel: [w295] -> w282
                              tunnel: [w295] -> w281 mode=indexing
                              tunnel: [w294] -> w279 mode=indexing
                              n207 = while {
                                tunnel: w303 -> [w324]
                                tunnel: w302 -> [w323]
                                tunnel: w301 -> [w321]
                                tunnel: w300 -> [w316]
                                tunnel: [w310] -> w299
                                tunnel: [w307] -> w298
                                tunnel: [w305] -> w296
                                tunnel: [w304] -> w294
                                i -> [w308]
                                stop <- w311 stop-if-true
                                n208 = property on="C1" class="DigNum (strict)"() -> ("Value"=w304:dbl)  [unwired: 2 in, 2 out]
                                n209 = property on="Mixed" class="Arr (strict)"() -> ("Value"=w322:dbl[])  [unwired: 2 in, 2 out]
                                n210 = Multiply(x=w316, y=1.01) -> (x*y=w318:dbl)
                                n211 = Multiply(x=w316, y=0.91) -> (x*y=w315:dbl)
                                n212 = Less?(x=10, y=w308) -> (x < y?=w320:bool)
                                n213 = call "ColorMixture.vi"("Concentration1"=w304, "Reflectance spectrum 2"=w323, "Reflectance spectrum"=w324) -> ("Mixtured colors"=w307:dbl[])  [unwired: 1 in]
                                n214 = call "SpectrumDeltaE.vi"("Iluminant - RGB - CMF"=w321, "Reflectance 2"=w322, "Reflectance 1"=w307) -> ("Color1"=w310:T4, "Delta E"=w305:dbl)  [unwired: 1 in, 1 out]
                                n215 = Greater?(x=w305, y=w318) -> (0:w309:bool)
                                n216 = Less?(x=w305, y=w315) -> (x < y?=w314:bool)
                                n217 = Or(x=w309, y=w314) -> (x .or. y?=w312:bool)
                                n218 = case shown="True" w312 {
                                tunnel: w305 -> [_ _]
                                tunnel: w309 -> [_ w325]
                                frame False {
                                }
                                frame True {
                                n219 = case shown="False" w325 {
                                frame False {
                                n220 = stacked-sequence {
                                frame #0 {
                                n221 = property on="C1" class="DigNum (strict)"() -> ("Value"=w326:dbl)  [unwired: 2 in, 2 out]
                                n222 = property on="C0" class="DigNum (strict)"("Value"=w326) -> ()  [unwired: 2 in, 2 out]
                                }
                                frame #1 {
                                n223 = property on="C1" class="DigNum (strict)"() -> ("Value"=w328:dbl)  [unwired: 2 in, 2 out]
                                n224 = formula code="C1=C1*1.5;\nif(C1 > 1)\nC1 = 0.99;"("C1"=w328) -> ("C1"=w327:dbl)
                                n225 = property on="C1" class="DigNum (strict)"("Value"=w327) -> ()  [unwired: 2 in, 2 out]
                                }
                                }
                                }
                                frame True {
                                n226 = property on="C0" class="DigNum (strict)"() -> ("Value"=w330:dbl)  [unwired: 2 in, 2 out]
                                n227 = property on="C1" class="DigNum (strict)"() -> ("Value"=w331:dbl)  [unwired: 2 in, 2 out]
                                n228 = formula code="C1 = (C1+C0)/2;\nif(C1 > 1)\nC1 = 0.99;"("C1"=w331, "C0"=w330) -> ("C1"=w329:dbl)
                                n229 = property on="C1" class="DigNum (strict)"("Value"=w329) -> ()  [unwired: 2 in, 2 out]
                                }
                                }
                                }
                                }
                                n230 = Not(x=w312) -> (.not. x?=w313:bool)
                                n231 = Or(x=w313, y=w320) -> (x .or. y?=w311:bool)
                              }
                              n232 = property on="Mixed" class="Arr (strict)"("Value"=w298) -> ()  [unwired: 2 in, 2 out]
                              n233 = Unbundle(w299) -> ("Color"=w297:u32, "L*a*b*"=w295:dbl[])  [unwired: 2 out]
                            }
                          }
                          frame #1 {
                            n234 = property on="Color1" class="DigNum (strict)"() -> ("Value"=w372:u32)  [unwired: 2 in, 2 out]
                            n235 = property on="Color2" class="DigNum (strict)"() -> ("Value"=w373:u32)  [unwired: 2 in, 2 out]
                            n236 = Unbundle By Name(w366) -> ("Color"=→"Color2 2":u32, "L*a*b*"=w339:dbl[])
                            n237 = Unbundle By Name(w365) -> ("Color"=→"Color1 2":u32, "L*a*b*"=w340:dbl[])
                            n238 = Insert Into Array(array=w361, index (row)=0, new element=w356) -> (w357:dbl[][])  [unwired: 1 in]
                            n239 = Insert Into Array(array=w357, index (row)=10, new element=w355) -> (w359:dbl[][])  [unwired: 1 in]
                            n240 = Number To Fractional String(number=w353, precision (6)=i16 2) -> (F-format string=w352:string[])  [unwired: 2 in]
                            n241 = call "BuildConcentrationString.vi"("Concentrations"=w333) -> ("Concentration String"=w332:string[])
                            n242 = Insert Into Array(array=w362, index=0, new element=w372) -> (w370:u32[])
                            n243 = Insert Into Array(array=w370, index=10, new element=w373) -> (w363:u32[])
                            n244 = property on="LambdaInterval" class="Arr (strict)"() -> ("Value"=w341:dbl[])  [unwired: 2 in, 2 out]
                            n245 = property on="Colors" class="Arr (strict)"("Value"=w363) -> ()  [unwired: 2 in, 2 out]
                            n246 = property on="ConcentrationLabel" class="Arr (strict)"("Value"=w332) -> ()  [unwired: 2 in, 2 out]
                            n247 = Insert Into Array(array=w352, index=0, new element="0" ("new element/subarray")) -> (w344:string[])
                            n248 = call "BuildGraph.vi"("X"=w341, "Y"=w359) -> ("Graph"=w364:cluster{"X":dbl[], "Y":dbl[]}[])
                            n249 = call "BuildLabDeltaGraph.vi"("L*a*b intermediary"=w338, "L*a*b 2"=w339, "L*a*b 1"=w340) -> ("L*a*b* Graphs"=w337:T6)
                            n250 = Bundle("L*a*b*"=w340, "L*a*b*"=w349) -> (w348:cluster{"L*a*b*":dbl[], "L*a*b*":dbl[]})  [unwired: 1 in]
                            n251 = property on="Espectros de reflectância referentes as cores intermediárias obtidas" class="XYGraph (strict)"("Value"=w364) -> ()  [unwired: 2 in, 2 out]
                            n252 = call "DeltaE(2000).vi"("L*a*b Colors"=w348) -> ("Delta E"=w346:dbl)
                            n253 = Number To Fractional String(number=w346, precision (6)=i16 2) -> (F-format string=w342:string)  [unwired: 2 in]
                            n254 = Insert Into Array(array=w344, index=10, new element=w342) -> (w343:string[])
                            n255 = property on="DeltaLabel" class="Arr (strict)"("Value"=w343) -> ()  [unwired: 2 in, 2 out]
                            n256 = Unbundle(w337) -> (w336:cluster{"X":dbl[], "L*a*b intermediary":dbl[]}, w335:cluster{"X":dbl[], "L*a*b intermediary":dbl[]}, w334:cluster{"X":dbl[], "L*a*b intermediary":dbl[]})
                            n257 = property on="Componente L*" class="XYGraph (strict)"("Value"=w336) -> ()  [unwired: 2 in, 2 out]
                            n258 = property on="Componente b*" class="XYGraph (strict)"("Value"=w335) -> ()  [unwired: 2 in, 2 out]
                            n259 = property on="Componente a*" class="XYGraph (strict)"("Value"=w334) -> ()  [unwired: 2 in, 2 out]
                          }
                        }
                      }
                    }
                  }
                }
              }
            }
          }
        }
        n260 = Wait (ms)(milliseconds to wait=u32 150) -> ()  [unwired: 1 out]
      }
    }
  }
  n261 = case shown="False" FALSE {
    frame False {
    }
    frame True {
      n262 = stacked-sequence {
        frame #0 {
          n263 = for {
            N: 81 -> [_]
            tunnel: [0] -> w403 mode=indexing
          }
          "teste" <- w403
        }
        frame #1 {
          n264 = for {
            N: 81 -> [_]
            i -> [w411]
            n265 = property on="Selected illuminant value" class="Arr (strict)"() -> ("Value"=w409:dbl[])  [unwired: 2 in, 2 out]
            n266 = property on="teste" class="Arr (strict)"() -> ("Value"=w410:i32[])  [unwired: 2 in, 2 out]
            n267 = Insert Into Array(array=w410, index=w411, new element=1 ("new element/subarray")) -> (w408:i32[])
            n268 = property on="Selected\nCMF" class="Arr (strict)"() -> ("Value"=w407:dbl[][])  [unwired: 2 in, 2 out]
            n269 = call "CalculateXYZ.vi"("CMF"=w407, "Reflectance"=w408, "Illuminant"=w409) -> ()  [unwired: 1 out]
          }
        }
      }
    }
  }
